vi "SwerveDrivePoseEst2_Pack_Config.vi"(5 "Wheel_Locations M":T1[](array[typedef]) {"Y" format="%14.3f"; "X" format="%14.3f"}, 6 "Vision Heading std dev Rad":dbl=0.9, 7 "Odom X std dev M":dbl=0.1, 8 "Vision Y std dev M":dbl=0.9, 9 "Vision X std dev M":dbl=0.9, 10 "Odom Heading std dev Rad":dbl=0.1, 11 "Odom Y std dev M":dbl=0.1) -> (3 "SwervePoseEst2Config":T2={"Wheel_Locations M"=[], "Odom X std dev M"=0.02, "Odom Y std dev M"=0.02, "Odom Heading std dev Rad"=0.01, "Vision X std dev M"=0.1, "Vision Y std dev M"=0.1, "Vision Heading std dev Rad"=0.05} {"Vision Heading std dev Rad" format="%#_13g"; "Vision Y std dev M" format="%#_13g"; "Vision X std dev M" format="%#_13g"; "Odom Heading std dev Rad" format="%#_13g"; "Odom Y std dev M" format="%#_13g"; "Odom X std dev M" format="%#_13g"; "Wheel_Locations M"."Y" format="%14.3f"; "Wheel_Locations M"."X" format="%14.3f"})   [LabVIEW 2019, in "Trajectory_Library.lvlib"]
doc: "Pack indvidual values into the cluster required by the SwerveDrivePoseEst2_Execute function. \n\nInputs\n - Wheel Locations M -- Translation2d array -- Locations of module wheels in relation to center of robot. (meters)\n - Odom X Std Dev M -- double -- Odometry X position standard deviation (Default: 0.02) (meters)\n - Odom Y Std Dev M -- double -- Odometry Y position standard deviation (Default: 0.02) (meters)\n - Odom Heading Std Dev M -- double -- Odometry Heading (gyro) position standard deviation (Default: 0.01) (radians)\n - Vision X Std Dev M -- double -- Vision X position standard deviation (Default: 0.1) (meters)\n - Vision Y Std Dev M -- double -- Vision Y position standard deviation (Default: 0.1) (meters)\n - Vision Heading Std Dev M -- double -- Vision Heading (gyro) position standard deviation (Default: 0.05) (radians)\n\nOutputs:\n - SwervePoseEst2Config -- cluster -- Packed data values."
uses:
  Trajectory_Library.lvlib
  TypeDef/SWERVE_DRIVE_POSE_EST2_CONFIG.ctl
  TypeDef/TRANSLATION2D.ctl
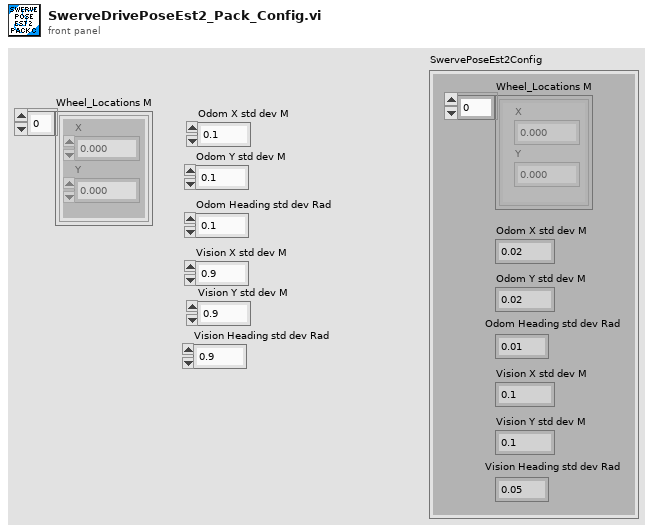
[diagram p1: front panel]
types:
  T1 = typedef "Trajectory_Library.lvlib/TRANSLATION2D.ctl" = cluster{"X":dbl, "Y":dbl}
  T2 = typedef "Trajectory_Library.lvlib/SWERVE_DRIVE_POSE_EST2_CONFIG.ctl" = cluster{"Wheel_Locations M":T1[], "Odom X std dev M":dbl, "Odom Y std dev M":dbl, "Odom Heading std dev Rad":dbl, "Vision X std dev M":dbl, "Vision Y std dev M":dbl, "Vision Heading std dev Rad":dbl}
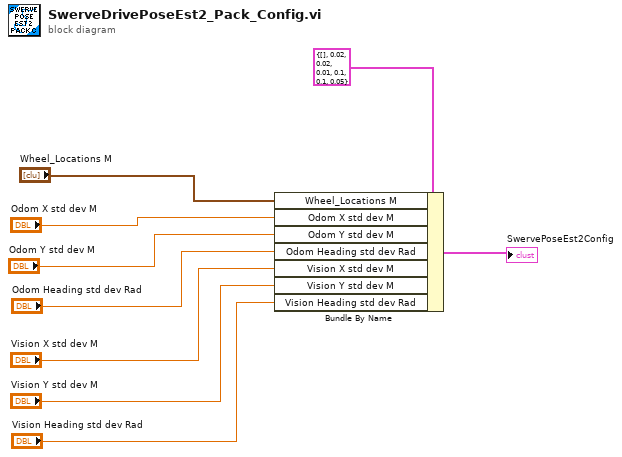
[diagram p0: block diagram]
diagram:
  n1 = Bundle By Name(cluster=T2 {"Wheel_Locations M"=[], "Odom X std dev M"=0.02, "Odom Y std dev M"=0.02, "Odom Heading std dev Rad"=0.01, "Vision X std dev M"=0.1, "Vision Y std dev M"=0.1, "Vision Heading std dev Rad"=0.05} ("SwervePoseEst2Config"), "Wheel_Locations M"="Wheel_Locations M", "Odom X std dev M"="Odom X std dev M", "Odom Y std dev M"="Odom Y std dev M", "Odom Heading std dev Rad"="Odom Heading std dev Rad", "Vision X std dev M"="Vision X std dev M", "Vision Y std dev M"="Vision Y std dev M", "Vision Heading std dev Rad"="Vision Heading std dev Rad") -> (→"SwervePoseEst2Config":T2)
